vi "Initial Values-Unbundler-DBL.vi"(8 "error in (no error)":errorcluster, 9 "Keys Array":T2, 10 "Section name":string, 11 "User profile ini file ref":T1) -> (0 "error out":errorcluster, 3 "User profile ini file ref":T1)   [LabVIEW 2020]
uses:
  Typedefs/Ini file interface (DBL).ctl
  <vilib>/Utility/config.llb/Config Data RefNum.ctl
  User Interface/Visualisation/Functional Imaging Viewer/Typedefs/Get-Set-Clear Control.ctl
  User Interface/Visualisation/Timelapse Viewer/Globals/gl_Time series viewer globals.vi
  Global Variables/gl_UI Ctrl Refs.vi
  <vilib>/Utility/config.llb/NI_LVConfig.lvlib
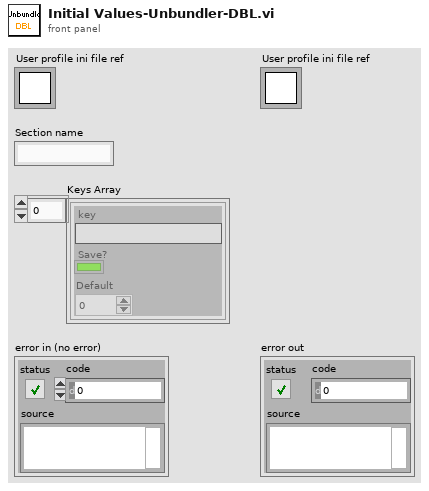
[diagram p1: front panel]
types:
  T1 = typedef "NI_LVConfig.lvlib/Config Data RefNum.ctl" = refnum<k1>
  T2 = typedef "Ini file interface (DBL).ctl" = cluster{"key":string, "Save?":bool, "Default":dbl}[]
  T3 = typedef "Get-Set-Clear Control.ctl" = enum16{"Get", "Set", "Clear"}
  T4 = typedef "UI ctrl refs cluster.ctl" = cluster{"Top level VI path":path, "Top level VI ref":refnum<vi>, "User menu ref":refnum<k9>, "Sub Panel control":refnum<vi>, "Imaging Param Tab":refnum<vi>, "Occurrence-Start drivers":refnum<k4>, "Occurrence-Speed logging initialised":refnum<k4>, "Occurrence-XYZ stage initialised":refnum<k4>, "Exit button":refnum<vi>, "Status ind":refnum<vi>, "Set as origin":refnum<vi>, "Speed Logging":refnum<vi>, "Time Lapse":refnum<vi>, "Live Imaging":refnum<vi>, "AOL Z Stack":refnum<vi>, "Motor Z Stack":refnum<vi>, "Funct Acq button":refnum<vi>, "Hard Shutter":refnum<vi>, "Virtual Shutter":refnum<vi>, "Laser Power":refnum<vi>, "AOL Mode":refnum<vi>, "Frame Size":refnum<vi>, "Field of View":refnum<vi>, "Dwell Time":refnum<vi>, "Zoom":refnum<vi>, "AOL Z":refnum<vi>, "Objective":refnum<vi>, "Axis":refnum<vi>, "Paths & Names":refnum<vi>, "Experiment folder path (ind.)":refnum<vi>, "Last State (Ind.)":refnum<vi>, "Averages":refnum<vi>, "Angle (degrees)":refnum<vi>, "X centre":refnum<vi>, "Y centre":refnum<vi>, "Plane Mode":refnum<vi>, "# Planes":refnum<vi>, "Z Start":refnum<vi>, "Z Stop":refnum<vi>, "Z Step":refnum<vi>, "PMT 1":refnum<vi>, "PMT 2":refnum<vi>, "Stage XYZ Position":refnum<vi>, "Pockels@Z Start":refnum<vi>, "Pockels@Z Stop":refnum<vi>, "Obtain Z Start":refnum<vi>, "Obtain Z Stop":refnum<vi>, "Live stim.trig.period":refnum<vi>, "Live stim.trig.enable":refnum<vi>, "Movement Correction":refnum<vi>, "Load Reference Image":refnum<vi>, "XY Stage Move":refnum<vi>, "MovCor Cluster":refnum<vi>, "RefDAQParam":refnum<vi>, "Funct. Acq. Pockels Modulation":refnum<vi>, "Ref Laser Power":refnum<vi>, "Enable Video Recording":refnum<vi>, "Video Record-Live Imaging":refnum<vi>, "Video Record-Funct acq":refnum<vi>, "Reference Source":refnum<vi>, "AOL Z-stack Chirps Ready (ind)":refnum<vi>, "Target time between mov.cor. ref triggers (ms)":refnum<vi>, "Funct. Acq. Ref frame save":refnum<vi>, "Tracking button":refnum<vi>, "Show ref plots window":refnum<vi>, "Center freq ind (nm)":refnum<vi>, "Pickup mode (ind)":refnum<vi>, "Logging queue (ind)":refnum<vi>, "Back aperture power (ind.)":refnum<vi>, "Power after objective (ind.)":refnum<vi>, "Switch user":refnum<vi>, "Ls1 Conn. Status":refnum<vi>, "Ls1Tuning Status":refnum<vi>, "Ls1 Faults":refnum<vi>, "Ls1 Connection":refnum<vi>, "Ls1 Mode":refnum<vi>, "Ls1 POWER [mW]":refnum<vi>, "Ls1Shutter":refnum<vi>, "Ls1 Wavelength":refnum<vi>, "Ls1 Note":refnum<vi>, "Ls1 Confirm Wav":refnum<vi>, "Ls1 PreChrp Prism1":refnum<vi>, "Ls1 PreChrp Prism2":refnum<vi>, "Ls1 wav top Ind":refnum<vi>, "Ls1 power top Ind":refnum<vi>, "Ls1 Pump peak Hold":refnum<vi>, "Ls1 Status Ind":refnum<vi>, "Ls1 wav cancel":refnum<vi>, "Experiment Type":refnum<vi>, "Biology Information":refnum<vi>, "Camera recording status":refnum<vi>}
  T5 = typedef "AOL_Globals.ctl" = cluster{"Imaging Protocol":T6, "Number of POI":u16, "Number of Miniscans":u16, "Number of Trials":u16, "Number of Cycles ":u64, "# Averaged Frames":u16, "Laser power (%)":u8, "Pockels (V)":dbl, "Acquisition Length (sec)":dbl, "Fill time (us)":dbl, "POI Dwell time (us)":dbl, "Miniscan Dwell time per pixel (us)":dbl, "PMT 1":dbl, "PMT 2":dbl, "Back Apperture (mA)":dbl, "Frame Size":T7, "Center Frequency":dbl, "Field of View (norm)":dbl, "DwellTime (us)":dbl, "Wavelength (nm)":dbl, "Zoom":dbl, "AOL Z":dbl, "AOL Mode":T8, "GridXY":dbl, "GridZ":dbl, "TriggerPeriod (sec)":dbl, "Number of Pixels in Miniscan":u16, "Experiment folder path":path, "X centre":dbl, "Y centre":dbl, "Angle (degrees)":dbl, "Plane Mode":T9, "Threshold":u16[], "Regenerate Chirps":bool, "Rectangle ROI length (pixels)":u16, "Rectangle ROI height (pixels)":u16, "AOD fill":u16, "StartupDelay":i32, "Samples Wait after Trigger":u16, "Slip Cycle":u32, "Add Cycle":bool, "Functional Mode":T10, "Z Start":dbl, "Z Stop":dbl, "# Planes":i32, "Total Pixels":i32, "Variable Miniscan Pixels":u16[], "Use Variable Length":bool, "Use Variable Resolution":bool, "Laser power (%) at Z Start":u8, "Laser power (%) at Z Stop":u8, "Ref Z Step":i8, "Ref Dwell Time (us)":dbl, "Field of View (um)":dbl}
  T6 = typedef "Imaging Protocols enum.ctl" = enum16{"AOL Z-Stack", "Motor Z Stack", "Functional Acquisition", "Single Plane Acquisition", "Volume Acquisition", "Live Imaging", "Live Plane Imaging", "Live Volume Imaging"}
  T7 = typedef "Frame Size.ctl" = u16
  T8 = typedef "AOL modes.ctl" = enum16{"Raster", "Structural", "Pointing", "Mini Scan", "Alignment"}
  T9 = typedef "Plane Mode.ctl" = u16
  T10 = typedef "Functional Mode.ctl" = enum16{"Point", "Line", "Patch", "Plane", "Volume"}
  T11 = typedef "Stitch layout spec cluster.ctl" = cluster{"Timelapse image":cluster{"Image position":T12}, "Cam 1":cluster{"Image position":T12}, "Cam 2":cluster{"Image position":T12}, "Cam 3":cluster{"Image position":T12}, "Cam 4":cluster{"Image position":T12}}
  T12 = typedef "Image stitching positions.ctl" = enum16{"Top left", "Top right", "Bottom left", "Bottom right", "Not used"}
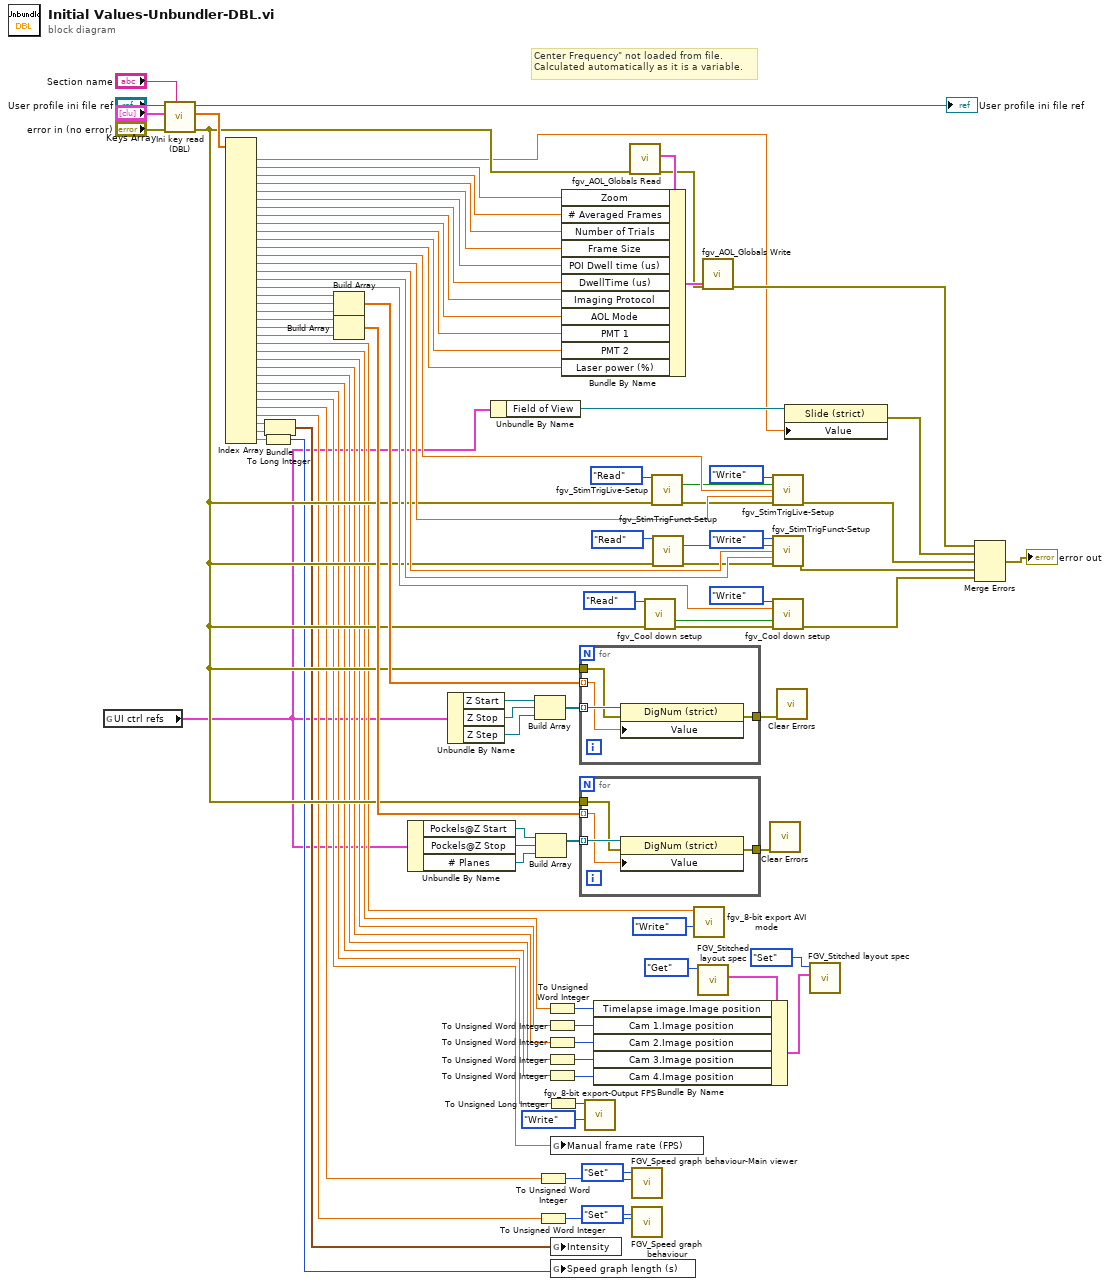
[diagram p0: block diagram]
diagram:
  # "Center Frequency\" not loaded from file.\nCalculated automatically as it is a variable."
  n1 = global read "gl_UI Ctrl Refs.vi" "UI ctrl refs"() -> (w5:T4)
  n2 = call "Ini key read (DBL).vi"("Section name"="Section name", "error in (no error)"="error in (no error)", "Parameter names & setup"="Keys Array", "Ini file refnum in"="User profile ini file ref") -> ("error out"=w42:errorcluster, "Value read/used"=w67:dbl[], "Ini file refnum out"=→"User profile ini file ref":T1)  [unwired: 5 in]
  n3 = Index Array(array=w67) -> (element #1=w2:dbl, element #2=w84:dbl, element #3=w85:dbl, element #4=w86:dbl, element #5=w87:dbl, element #6=w88:dbl, element #7=w89:dbl, element #8=w90:dbl, element #9=w91:dbl, element #10=w92:dbl, element #11=w83:dbl, element #12=w82:dbl, element #13=w81:dbl, element #14=w80:dbl, element #15=w79:dbl, element #16=w78:dbl, element #17=w96:dbl, element #18=w56:dbl, element #19=w55:dbl, element #20=w54:dbl, element #21=w52:dbl, element #22=w51:dbl, element #23=w39:dbl, element #24=w26:dbl, element #25=w25:dbl, element #26=w24:dbl, element #27=w23:dbl, element #28=w22:dbl, element #29=w21:dbl, element #30=w20:dbl, element #31=w19:dbl, element #32=w16:dbl, element #33=w15:dbl, element #34=w10:dbl, element #35=w9:dbl, element #36=w7:dbl)  [unwired: 36 in]
  n4 = To Long Integer(number=w7) -> (32bit integer=w6:i32)
  n5 = Bundle("value"=w10, "value"=w9) -> (w8:cluster{"value":dbl, "value":dbl})  [unwired: 1 in]
  n6 = Build Array(w56, w55, w54) -> (w53:dbl[])
  n7 = Build Array(w52, w51, w39) -> (w50:dbl[])
  n8 = Unbundle By Name(w5) -> ("Pockels@Z Start"=w58:refnum<vi>, "Pockels@Z Stop"=w59:refnum<vi>, "# Planes"=w40:refnum<vi>)
  n9 = Unbundle By Name(w5) -> ("Z Start"=w63:refnum<vi>, "Z Stop"=w61:refnum<vi>, "Z Step"=w60:refnum<vi>)
  n10 = Unbundle By Name(w5) -> ("Field of View"=w4:refnum<vi>)
  n11 = Build Array(w63, w61, w60) -> (w62:refnum<vi>[])
  n12 = Build Array(w58, w59, w40) -> (w57:refnum<vi>[])
  n13 = To Unsigned Word Integer(number=w16) -> (unsigned 16bit integer=w12:u16)
  n14 = To Unsigned Word Integer(number=w15) -> (unsigned 16bit integer=w11:u16)
  n15 = To Unsigned Word Integer(number=w25) -> (unsigned 16bit integer=w34:u16)
  n16 = To Unsigned Word Integer(number=w24) -> (unsigned 16bit integer=w33:u16)
  n17 = To Unsigned Word Integer(number=w23) -> (unsigned 16bit integer=w32:u16)
  n18 = To Unsigned Word Integer(number=w22) -> (unsigned 16bit integer=w31:u16)
  n19 = To Unsigned Word Integer(number=w21) -> (unsigned 16bit integer=w30:u16)
  n20 = To Unsigned Long Integer(number=w20) -> (unsigned 32bit integer=w27:u32)
  n21 = global write "gl_Time series viewer globals.vi" "Manual frame rate (FPS)"(w19) -> ()
  n22 = global write "gl_Time series viewer globals.vi" "Intensity"(w8) -> ()
  n23 = global write "gl_Time series viewer globals.vi" "Speed graph length (s)"(w6) -> ()
  n24 = for {
    tunnel: w62 -> [w100] mode=indexing
    tunnel: w53 -> [w99] mode=indexing
    tunnel: [w98] -> w18
    tunnel: w42 -> [w97]
    n25 = property class="DigNum (strict)"(reference=w100, error in=w97, "Value"=w99) -> (error out=w98:errorcluster)  [unwired: 1 out]
  }
  n26 = for {
    tunnel: w57 -> [w104] mode=indexing
    tunnel: w50 -> [w103] mode=indexing
    tunnel: [w102] -> w17
    tunnel: w42 -> [w101]
    n27 = property class="DigNum (strict)"(reference=w104, error in=w101, "Value"=w103) -> (error out=w102:errorcluster)  [unwired: 1 out]
  }
  n28 = call "fgv_8-bit export-Output FPS.vi"("Function"=enum16{"Intialize", "Write", "Read", "Clear"}."Write", "Frames Per Second"=w27) -> ()  [unwired: 8 in, 2 out]
  n29 = call "fgv_AOL_Globals Read.vi"("error in (no error)"=w42) -> ("error out"=w49:errorcluster, "AOL_Globals"=w77:T5)  [unwired: 8 in, 1 out]
  n30 = Bundle By Name(cluster=w77, "Zoom"=w84, "# Averaged Frames"=w85, "Number of Trials"=w86, "Frame Size"=w87, "POI Dwell time (us)"=w88, "DwellTime (us)"=w89, "Imaging Protocol"=w90, "AOL Mode"=w91, "PMT 1"=w92, "PMT 2"=w83, "Laser power (%)"=w82) -> (w70:T5)
  n31 = call "FGV_Speed graph behaviour-Main viewer.vi"("Function"=Get-Set-Clear_Control."Set", "Speed graph behaviour"=w12) -> ()  [unwired: 8 in, 2 out]
  n32 = call "FGV_Speed graph behaviour.vi"("Function"=Get-Set-Clear_Control."Set", "Speed graph behaviour"=w11) -> ()  [unwired: 8 in, 2 out]
  n33 = call "fgv_Cool down setup.vi"("Function"=enum16{"Intialize", "Write", "Read", "Clear"}."Read", "error in (no error)"=w42) -> ("Enable cool-down time"=w95:bool, "error out"=w45:errorcluster)  [unwired: 11 in, 1 out]
  n34 = call "fgv_StimTrigLive-Setup.vi"("Function"=enum16{"Intialize", "Write", "Read", "Clear"}."Read", "error in (no error)"=w42) -> ("Live stim.trig.enable"=w73:bool, "error out"=w43:errorcluster)  [unwired: 10 in, 2 out]
  n35 = call "fgv_StimTrigFunct-Setup.vi"("Function"=enum16{"Intialize", "Write", "Read", "Clear"}."Read", "error in (no error)"=w42) -> ("Funct stim.trig.enable"=w76:bool, "error out"=w44:errorcluster)  [unwired: 10 in, 2 out]
  n36 = call "fgv_8-bit export AVI mode.vi"("Function"=enum16{"Intialize", "Write", "Read", "Clear"}."Write", "AVI mode"=w26) -> ()  [unwired: 8 in, 2 out]
  n37 = call "FGV_Stitched layout spec.vi"("Function"=Get-Set-Clear_Control."Get") -> ("Stitch layout spec"=w36:T11)  [unwired: 9 in, 1 out]
  n38 = Bundle By Name(cluster=w36, "Timelapse image.Image position"=w34, "Cam 1.Image position"=w33, "Cam 2.Image position"=w32, "Cam 3.Image position"=w31, "Cam 4.Image position"=w30) -> (w37:T11)
  n39 = call "fgv_AOL_Globals Write.vi"("error in (no error)"=w49, "AOL_Globals"=w70) -> ("error out"=w46:errorcluster)  [unwired: 9 in]
  n40 = call <vilib>:"Clear Errors.vi"("error in (no error)"=w17) -> ()  [unwired: 5 in, 2 out]
  n41 = call "fgv_StimTrigLive-Setup.vi"("Function"=enum16{"Intialize", "Write", "Read", "Clear"}."Write", "Live stim.trig.enable"=w73, "Live stim.trig.period (sec)"=w81, "Live stim.trig.width (ms)"=w80, "error in (no error)"=w43) -> ("error out"=w3:errorcluster)  [unwired: 7 in, 3 out]
  n42 = call "fgv_StimTrigFunct-Setup.vi"("Function"=enum16{"Intialize", "Write", "Read", "Clear"}."Write", "Funct stim.trig.enable"=w76, "Funct stim.trig.delay (sec)"=w79, "Funct stim.trig.width (ms)"=w78, "error in (no error)"=w44) -> ("error out"=w47:errorcluster)  [unwired: 7 in, 3 out]
  n43 = call "fgv_Cool down setup.vi"("Function"=enum16{"Intialize", "Write", "Read", "Clear"}."Write", "Cool-down time (s)"=w96, "Enable cool-down time"=w95, "error in (no error)"=w45) -> ("error out"=w48:errorcluster)  [unwired: 9 in, 2 out]
  n44 = call <vilib>:"Clear Errors.vi"("error in (no error)"=w18) -> ()  [unwired: 5 in, 2 out]
  n45 = property class="Slide (strict)"(reference=w4, "Value"=w2) -> (error out=w1:errorcluster)  [unwired: 1 in, 1 out]
  n46 = call "FGV_Stitched layout spec.vi"("Stitch layout spec"=w37, "Function"=Get-Set-Clear_Control."Set") -> ()  [unwired: 8 in, 2 out]
  n47 = Merge Errors(w46, w1, w3, w47, w48) -> (→"error out":errorcluster)
